vi "Get All Incoming Frames.vi"(8 "error in":errorcluster, 11 "Item Ref":T4 format="%.0x") -> (0 "error out":errorcluster, 2 "Frames":T3(array[cluster]) {"Frame Transmit Info"."Transmit Time" format="%#_p"}, 3 "Item Ref out":T4 format="%.0x")   [LabVIEW 2015, in "J1939 Addon System Explorer.lvlib"]
uses:
  J1939 Addon System Explorer.lvlib
  <vilib>/NI Veristand/Custom Device API/Custom Device Item Ref.ctl
  Shared/Types/XNET Frame Event Properties.ctl
  Shared/Types/SPN Properties.ctl
  Shared/SubVIs/Constants.vi
  <vilib>/NI Veristand/Custom Device Tools/Custom Device Utility Library/NI VeriStand - Search for All Items by GUID.vi
  <vilib>/NI Veristand/Custom Device API/Get Item Property (U32).vi
  <vilib>/NI Veristand/Custom Device API/Get Item Property (Variant).vi
  Shared/J1939 Addon Shared.lvlib
  <vilib>/NI Veristand/Custom Device Tools/Custom Device Utility Library/Custom Device Utility Library.lvlib
  <vilib>/NI Veristand/Custom Device API/Custom Device API.lvlib
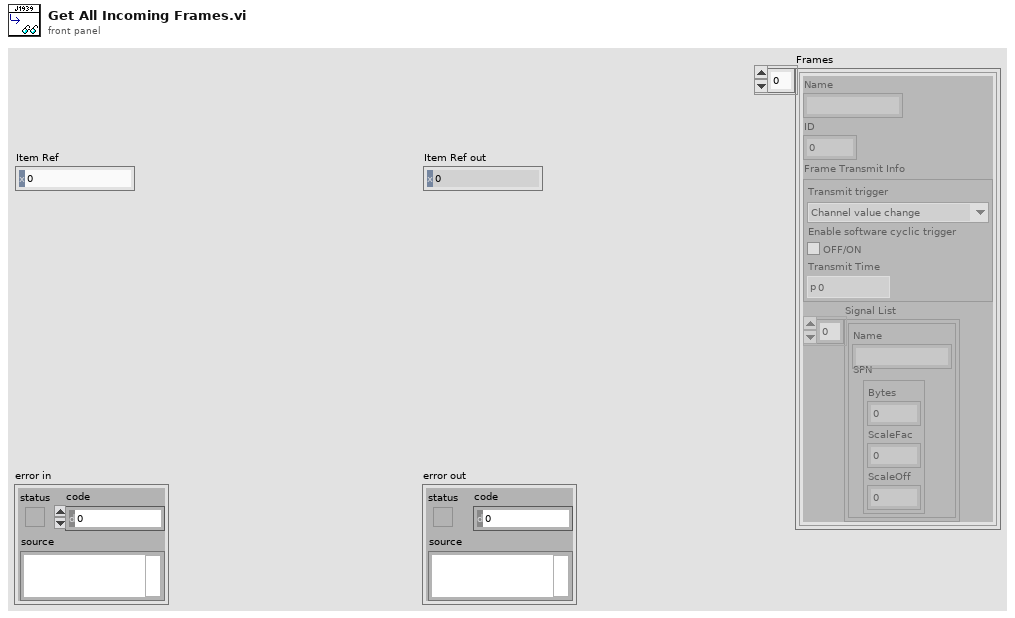
[diagram p1: front panel]
types:
  T1 = typedef "J1939 Addon Shared.lvlib/XNET Frame Event Properties.ctl" = cluster{"Transmit trigger":enum16{"Channel value change"}, "Enable software cyclic trigger":bool, "Transmit Time":dbl}
  T2 = typedef "J1939 Addon Shared.lvlib/SPN Properties.ctl" = cluster{"Bytes":u32, "ScaleFac":dbl, "ScaleOff":dbl}
  T3 = cluster{"Name":string, "ID":u32, "Frame Transmit Info":T1, "Signal List":cluster{"Name":string, "SPN":T2}[]}[]
  T4 = typedef "Custom Device API.lvlib/Custom Device Item Ref.ctl" = u64
  T5 = typedef "Custom Device API.lvlib/Custom Device Item Info.ctl" = cluster{"Name":string, "Is Channel":bool, "GUID":string, "Is Waveform":bool}
  T6 = cluster{"Name":string, "Value":u32, "Transmit Properties":T1, cluster{"Name":string, "cluster":T2}[]}
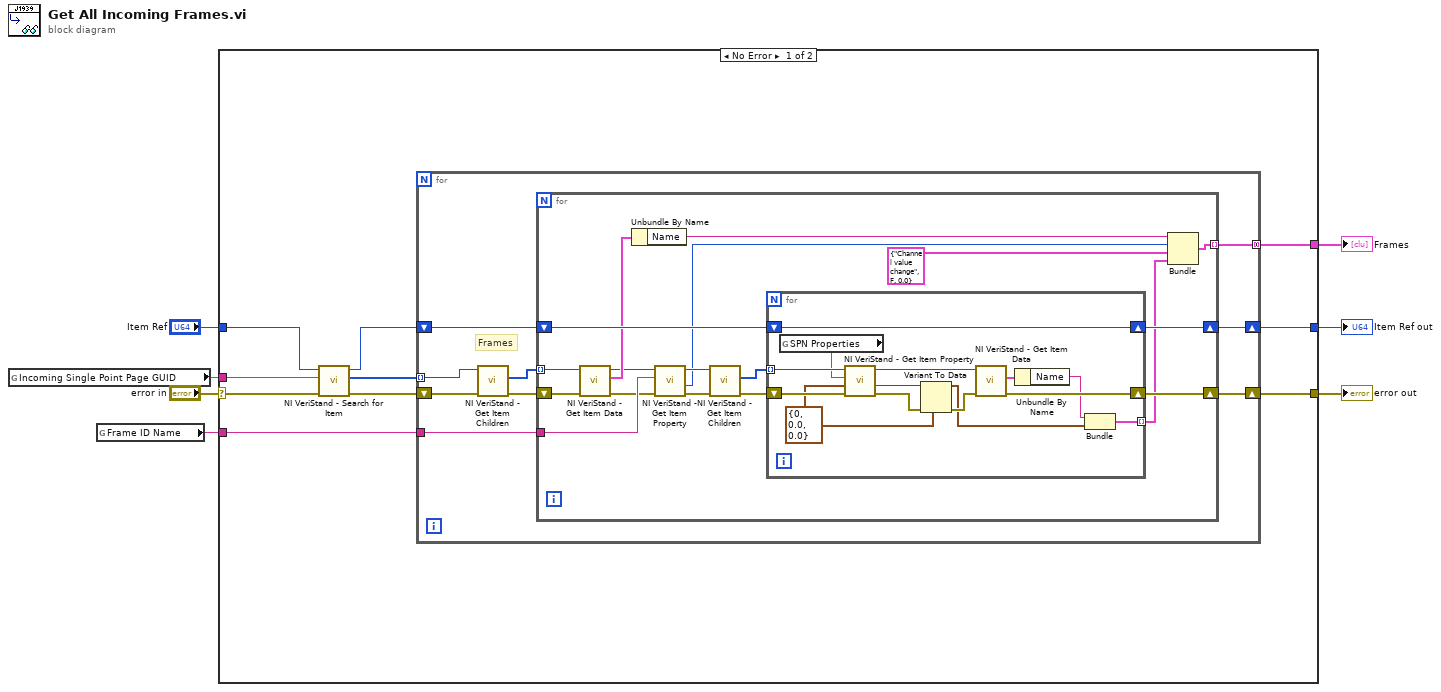
[diagram p0: block diagram]
diagram:
  n1 = global read "Constants.vi" "Incoming Single Point Page GUID"() -> (w3:string)
  n2 = global read "Constants.vi" "Frame ID Name"() -> (w6:string)
  n3 = case shown="No Error" "error in" {
    selector: "error in" -> [w12 w60]
    tunnel: [w14 w59] -> w7
    tunnel: w6 -> [w17 _]
    tunnel: [w13 w60] -> w5
    tunnel: "Item Ref" -> [w10 w59]
    tunnel: w3 -> [w11 _]
    tunnel: [w8 _] -> w1
    frame No Error {
      n4 = call-poly <vilib>:"NI VeriStand - Search for Item.vi"("error in"=w12, "Item GUID"=w11, "Section Ref in"=w10) -> ("error out"=w16:errorcluster, "Item Refs"=w15:T4[], "Section Ref out"=w9:T4)  [unwired: 5 in, 1 out]
      n5 = for {
        tunnel: w17 -> [w26]
        tunnel: w15 -> [w23] mode=indexing
        tunnel: [w19] -> w8 mode=concatenating
        shift-right: [w22] -> w14
        shift-left: w9 -> [w18]
        shift-right: [w20] -> w13
        shift-left: w16 -> [w24]
        # "Frames"
        n6 = call <vilib>:"NI VeriStand - Get Item Children.vi"("error in (no error)"=w24, "Item Ref in"=w23) -> ("error out"=w21:errorcluster, "Child Refs"=w25:T4[])  [unwired: 6 in, 2 out]
        n7 = for {
          shift-right: [w31] -> w20
          shift-left: w21 -> [w36]
          tunnel: w25 -> [w37] mode=indexing
          tunnel: w26 -> [w44]
          shift-right: [w39] -> w22
          shift-left: w18 -> [w40]
          tunnel: [w32] -> w19 mode=indexing
          n8 = call <vilib>:"NI VeriStand - Get Item Data.vi"("error in (no error)"=w36, "Item Ref in"=w37) -> ("error out"=w33:errorcluster, "Item Info"=w35:T5, "Item Ref out"=w34:T4)  [unwired: 6 in, 1 out]
          n9 = Unbundle By Name(w35) -> ("Name"=w29:string)
          n10 = call-poly <vilib>:"NI VeriStand - Get Item Property.vi"("error in (no error)"=w33, "Property Name"=w44, "Item Ref in"=w34) -> ("error out"=w43:errorcluster, "Value"=w30:u32, "Item Ref out"=w42:T4)  [unwired: 5 in, 1 out]
          n11 = call <vilib>:"NI VeriStand - Get Item Children.vi"("error in (no error)"=w43, "Item Ref in"=w42) -> ("error out"=w41:errorcluster, "Child Refs"=w38:T4[])  [unwired: 6 in, 2 out]
          n12 = for {
            shift-right: [w55] -> w31
            shift-left: w41 -> [w50]
            tunnel: w38 -> [w58] mode=indexing
            shift-right: [w56] -> w39
            shift-left: w40 -> [w56]
            tunnel: [w47] -> w28 mode=indexing
            w46 = T2 {"Bytes"=0, "ScaleFac"=0.0, "ScaleOff"=0.0} ("cluster")
            n13 = global read "Constants.vi" "SPN Properties"() -> (w53:string)
            n14 = call-poly <vilib>:"NI VeriStand - Get Item Property.vi"("error in (no error)"=w50, "Default Value"=w46, "Property Name"=w53, "Item Ref in"=w58) -> ("error out"=w49:errorcluster, "Value"=w51:variant, "Item Ref out"=w54:T4)  [unwired: 4 in, 1 out]
            n15 = Variant To Data(error in=w49, type=w46, Variant=w51) -> (data=w45:T2, error out=w52:errorcluster)
            n16 = call <vilib>:"NI VeriStand - Get Item Data.vi"("error in (no error)"=w52, "Item Ref in"=w54) -> ("error out"=w55:errorcluster, "Item Info"=w57:T5)  [unwired: 6 in, 2 out]
            n17 = Unbundle By Name(w57) -> ("Name"=w48:string)
            n18 = Bundle("Name"=w48, "cluster"=w45) -> (w47:cluster{"Name":string, "cluster":T2})  [unwired: 1 in]
          }
          n19 = Bundle("Name"=w29, "Value"=w30, "Transmit Properties"=T1 {"Transmit trigger"=enum."Channel value change", "Enable software cyclic trigger"=FALSE, "Transmit Time"=0.0}, w28) -> (w32:T6)  [unwired: 1 in]
        }
      }
    }
    frame Error {
    }
  }
  "error out" <- w5
  "Item Ref out" <- w7
  "Frames" <- w1
